vi "segmentation of lipid droplet area.vi"(1 "Cluster":T1={"Window Size (32x32)"={10, 10}, "Method (Niblack)"=0, "Dev rng"=100.0, "DevFact"=1.0, "image lpf in"={"cut"=0.2000001000000001, "lpf"=FALSE, "odr"=2}, "shift"=[], "itr"=1} {"image lpf in"."cut" min=1e-07 max=0.4999 step=0.01 format="%_2g"; "DevFact" min=0.0 max=1.0 format="%.2f"; "Method (Niblack)" items=["Niblack", "Background Correction", "Sauvola"]; "Window Size (32x32)"."?" min=3 step=1; "Window Size (32x32)"."?" min=3 step=1}, 2 "cell mask":dbl[][](array[numeric]), 3 "img":dbl[][](array[numeric])) -> (0 "Image Pixels (U8)":u8[][](array[numeric]))   [LabVIEW 2018]
uses:
  <vilib>/vision/NI_Vision_Development_Module.lvlib
panel:
  out "mask1 3":dbl[][](graph)
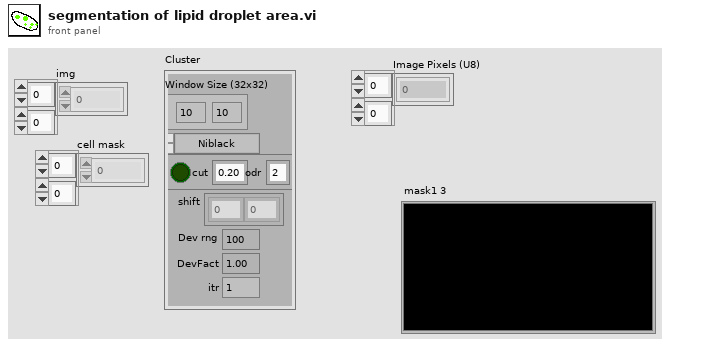
[diagram p1: front panel]
types:
  T1 = cluster{"Window Size (32x32)":cluster{i32, i32}, "Method (Niblack)":u32, "Dev rng":dbl, "DevFact":dbl, "image lpf in":cluster{"cut":dbl, "lpf":bool, "odr":i32}, "shift":i32[], "itr":i32}
  T2 = enum32{"AutoM", "Close", "Dilate", "Erode", "Gradient", "Gradient out", "Gradient in", "Hit miss", "Open", "PClose", "POpen", "Thick", "Thin"}
  T3 = typedef "Image Type" = u32
  T4 = typedef "IMAQ Image.ctl" = refnum<image>
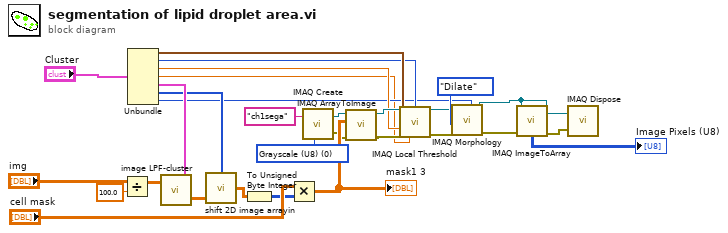
[diagram p0: block diagram]
diagram:
  w10 = T3 0 items=["Grayscale (U8)", "Grayscale (I16)", "Grayscale (SGL)", "Complex (CSG)", "RGB (U32)", "HSL (U32)", "RGB (U64)", "Grayscale (U16)"] ("Image Type")
  n1 = Divide(x="img", y=100.0) -> (x/y=w17:dbl[][])
  n2 = Unbundle("Cluster") -> ("Window Size (32x32)"=w7:cluster{i32, i32}, "Method (Niblack)"=w6:u32, "Dev rng"=w5:dbl, "DevFact"=w1:dbl, "image lpf in"=w4:cluster{"cut":dbl, "lpf":bool, "odr":i32}, "shift"=w3:i32[], "itr"=w2:i32)
  n3 = call "image LPF-cluster.vi"("image lpf"=w4, "input"=w17) -> ("output"=w18:dbl[][])  [unwired: 1 in]
  n4 = call "shift 2D image arrayin.vi"("Array in"=w18, "shift"=w3) -> ("Array out"=w19:dbl[][])
  n5 = To Unsigned Byte Integer(number=w19) -> (unsigned 8bit integer=w20:u8[][])
  n6 = Multiply(x="cell mask", y=w20) -> (x*y=w29:dbl[][])
  "mask1 3" <- w29
  n7 = call "IMAQ Create"("Image Name"="ch1sega", "Image Type"=w10) -> ("New Image"=w9:T4, "error out"=w11:errorcluster)  [unwired: 3 in]
  n8 = call "IMAQ ArrayToImage"("error in (no error)"=w11, "Image Pixels (U8)"=w29, "Image"=w9) -> ("error out"=w15:errorcluster, "Image Out"=w14:T4)  [unwired: 7 in]
  n9 = call "IMAQ Local Threshold"("Image Src"=w14, "Method (Niblack)"=w6, "Window Size (32x32)"=w7, "Sauvola Deviation Range"=w5, "error in (no error)"=w15, "Niblack/Sauvola Deviation Factor (0.2)"=w1) -> ("Image Dst Out"=w25:T4, "error out"=w23:errorcluster)  [unwired: 8 in]
  n10 = call "IMAQ Morphology"("Number of iterations (1)"=w2, "error in (no error)"=w23, "Operation"=T2."Dilate", "Image Src"=w25) -> ("error out"=w24:errorcluster, "Image Dst Out"=w26:T4)  [unwired: 6 in]
  n11 = call "IMAQ ImageToArray"("error in (no error)"=w24, "Image"=w26) -> ("error out"=w12:errorcluster, "Image Pixels (U8)"=→"Image Pixels (U8)":u8[][])  [unwired: 2 in, 3 out]
  n12 = call "IMAQ Dispose"("Image"=w26, "error in (no error)"=w12) -> ()  [unwired: 4 in, 1 out]
